vi "Scripting Mngr.vi"(0 "Path (dialog)":path, 1 "Mngr Action":T5, 3 "Main References":T4, 5 "Bottle X":T3, 7 "Drain X":T2, 9 "Well X":T1, 11 "error in (no error)":errorcluster, 12 "Script Choice":T6) -> (4 "selected path":path, 15 "error out":errorcluster)   [LabVIEW 2020]
uses:
  Script Mngr Script choice.ctl
  Script Mngr Action.ctl
  Main Refs.ctl
  Lib/Time/Bottles.ctl
  Drain Valve.ctl
  Lib/Time/Wells.ctl
  Hardware/Tricon Mngr.ctl
  Hardware/Tecan/Pump Control.ctl
  Pump Port.ctl
  Hardware/Tecan/Velocity Units.ctl
  Hardware/Valco Valve/Valco Valve Mngr Action.ctl
  Hardware/16CH Denkovi Mngr.ctl
  Hardware/Mot Stage Mngr.ctl
  Main Globals.vi
panel:
  in  "Pressure Valves X":bool[](array[boolean])
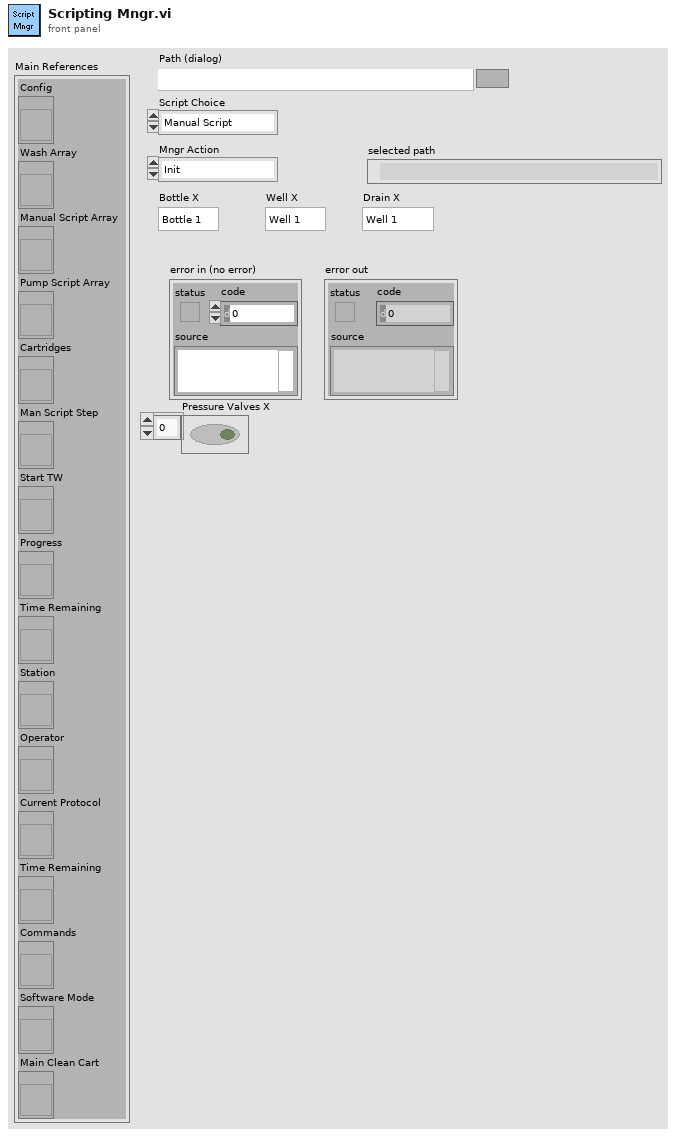
[diagram p1: front panel]
types:
  T1 = typedef "Wells.ctl" = enum16{"Well 1", "Well 2", "Well 3", "Well 4"}
  T2 = typedef "Drain Valve.ctl" = enum16{"Well 1", "Well 2", "Well 3", "Well 4", "Well X"}
  T3 = typedef "Bottles.ctl" = enum16{"Bottle 1", "Bottle 2", "Bottle 3", "H2O", "Waste"}
  T4 = typedef "Main Refs.ctl" = cluster{"Config":refnum<vi>, "Wash Array":refnum<vi>, "Manual Script Array":refnum<vi>, "Pump Script Array":refnum<vi>, "Cartridges":refnum<vi>, "Man Script Step":refnum<vi>, "Start TW":refnum<vi>, "Progress":refnum<vi>, "Time Remaining":refnum<vi>, "Station":refnum<vi>, "Operator":refnum<vi>, "Current Protocol":refnum<vi>, "Time Remaining":refnum<vi>, "Commands":refnum<vi>, "Software Mode":refnum<vi>, "Main Clean Cart":refnum<vi>}
  T5 = typedef "Script Mngr Action.ctl" = enum16{"Init", "Run Script", "Load Script", "Save Script", "Close"}
  T6 = typedef "Script Mngr Script choice.ctl" = enum16{"Manual Script", "Pump Script", "Wash Setup"}
  T7 = typedef "Pump Control.ctl" = cluster{"Syringe Pos":u32, "Rate":dbl, "Volume":dbl, "Valve":T8, "Action":enum32{"Withdraw", "Dispense", "Stop"}, "Move Type":enum32{"Abs", "Rel"}, "Init":bool, "Empty Syr.":bool, "Full Fill":bool, "Units":T9}
  T8 = typedef "Pump Port.ctl" = enum16{"Bottle 1", "Bottle 2", "Bottle 3", "Bottle 4", "Waste", "Well 1", "Well 2", "Well 3", "Well 4", "Bottle X", "Well X"}
  T9 = typedef "Velocity Units.ctl" = enum16{"ul/s", "ul/min"}
  T10 = typedef "Tricon Mngr.ctl" = enum16{"Init COM", "Set Config", "Init Pump", "Home", "Cmd", "Start Pump", "Set Valve", "Dispense", "Withdraw", "Status", "Close"}
  T11 = typedef "Mot Stage Mngr.ctl" = enum16{"Connect", "Init", "Status", "Send Cmd", "Current Pos", "Set Accel", "Set Max Vel", "Home", "Rel Move", "Abs Move", "Close"}
  T12 = typedef "16CH Denkovi Mngr.ctl" = enum16{"Search", "Init", "Set Peristaltic", "Set Pressure", "Set Vacuum", "Pres Vent&Close", "Vac Vent&Close", "Pres ON", "Vac ON", "Set All Relays", "Set One Relay", "Read Relays", "Close"}
  T13 = typedef "Valco Valve Mngr Action.ctl" = enum16{"Connect", "Init", "Cmd", "Set Valve", "Status", "Close"}
  T14 = typedef "Pump Script Step.ctl" = cluster{"Valve":enum16{"Valve 1", "Valve 2", "Valve 3", "Valve 4", "Valve 5", "Valve 6", "Valve 7", "Valve 8", "Valve 9"}, "Syr.Amount":dbl, "Syr.Rate":dbl, "move type":enum32{"rel", "abs"}, "direction":enum32{"withdraw", "dispense"}, "Delay(s)":dbl}
  T15 = enum16{"Valve 1", "Valve 2", "Valve 3", "Valve 4", "Valve 5", "Valve 6", "Valve 7", "Valve 8", "Valve 9"}
  T16 = typedef "Script Step.ctl" = cluster{"Step":dbl, "Step En":bool, "Valve":T8, "Syr.Amount":dbl, "Syr.Rate":dbl, "direction":enum32{"withdraw", "dispense"}, "Move Type":enum32{"Abs", "Rel"}, "Pump En":bool, "Drain Valve":T2, "Drain En":bool, "Peristaltic":bool, "Peristaltic En":bool, "Pres1":bool, "Pres2":bool, "Pres3":bool, "Pres4":bool, "Pressure En":bool, "Move Abs":dbl, "Motion En":bool, "Delay(s)":dbl, "Delay En":bool, "Use PresX":bool, "Vac1":bool, "Vac2":bool, "Vac3":bool, "Vac4":bool, "Use VacX":bool}
  T17 = typedef "Wash Step.ctl" = cluster{"Reagent":string, "Bottle":enum16{"Bottle 1", "Bottle 2", "Bottle 3", "Bottle 4"}, "Wash Time(s)":dbl, "Dwell Time(s)":dbl, "# of Rinses":i16}
  T18 = cluster{"negative limit switch":bool, "positive limit switch":bool, "home switch":bool, "position marker":bool, "device enable":bool, "quick stop":bool, "general purpose J":bool, "general purpose I":bool, "general purpose H":bool, "general purpose G":bool, "general purpose F":bool, "general purpose E":bool, "general purpose D":bool, "general purpose C":bool, "general purpose B":bool, "general purpose A":bool}
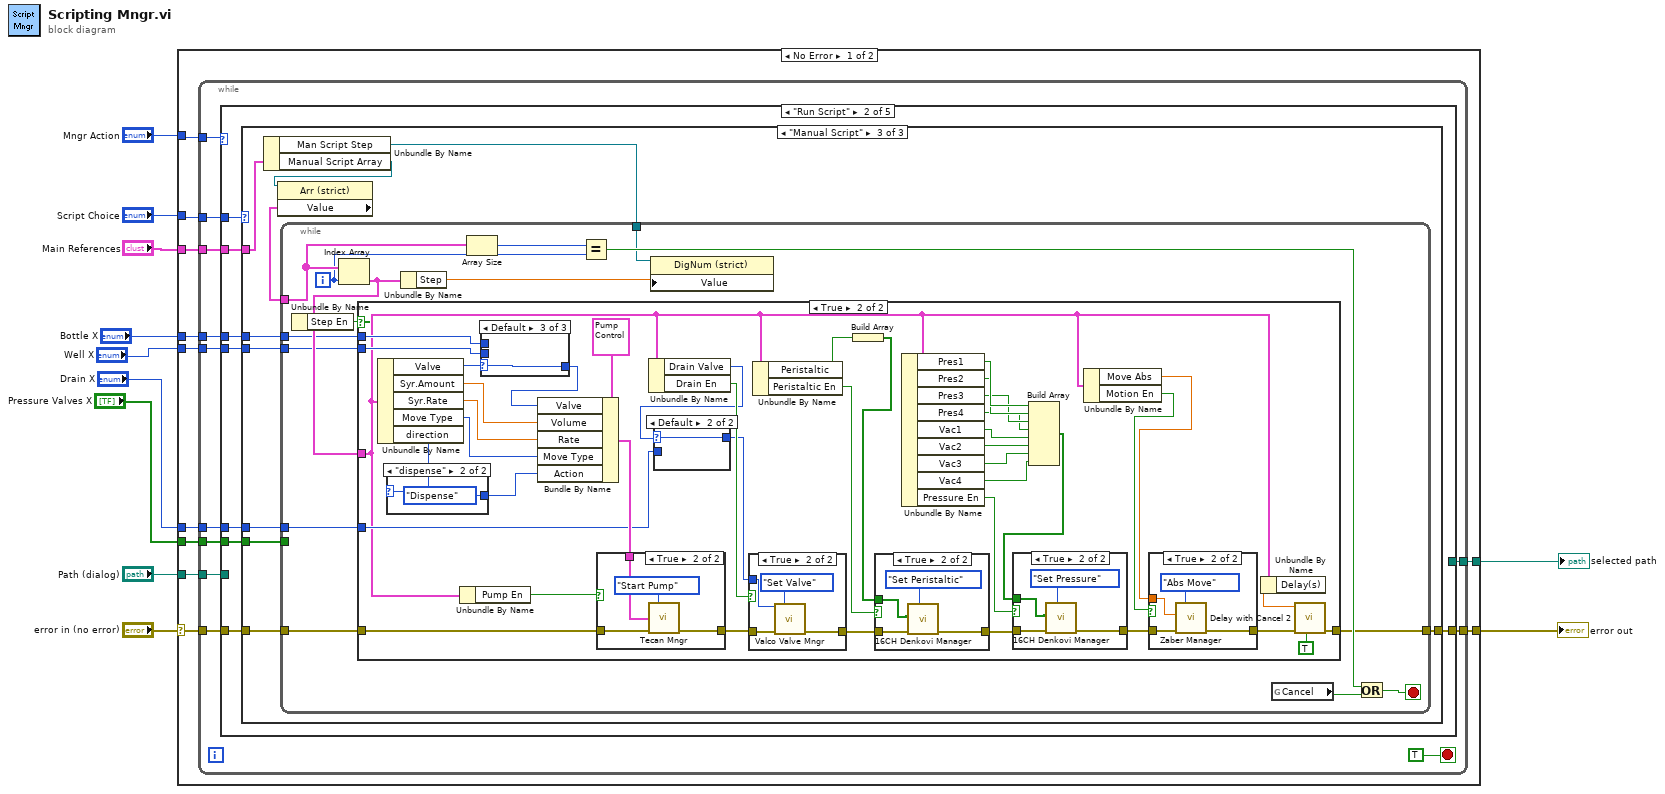
[diagram p0: block diagram]
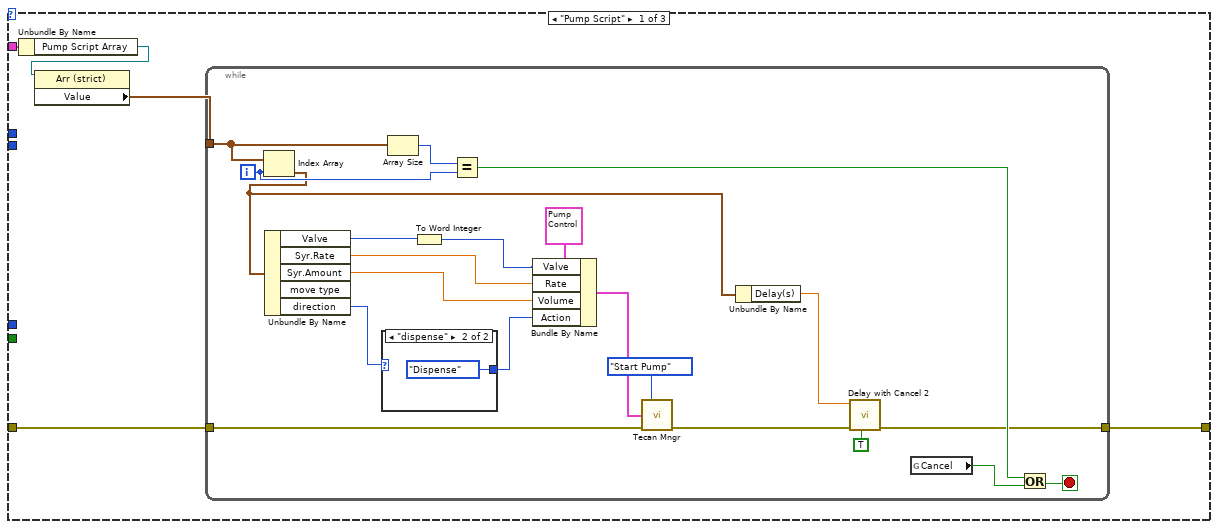
[diagram p3: hidden frame]
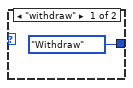
[diagram p4: hidden frame]
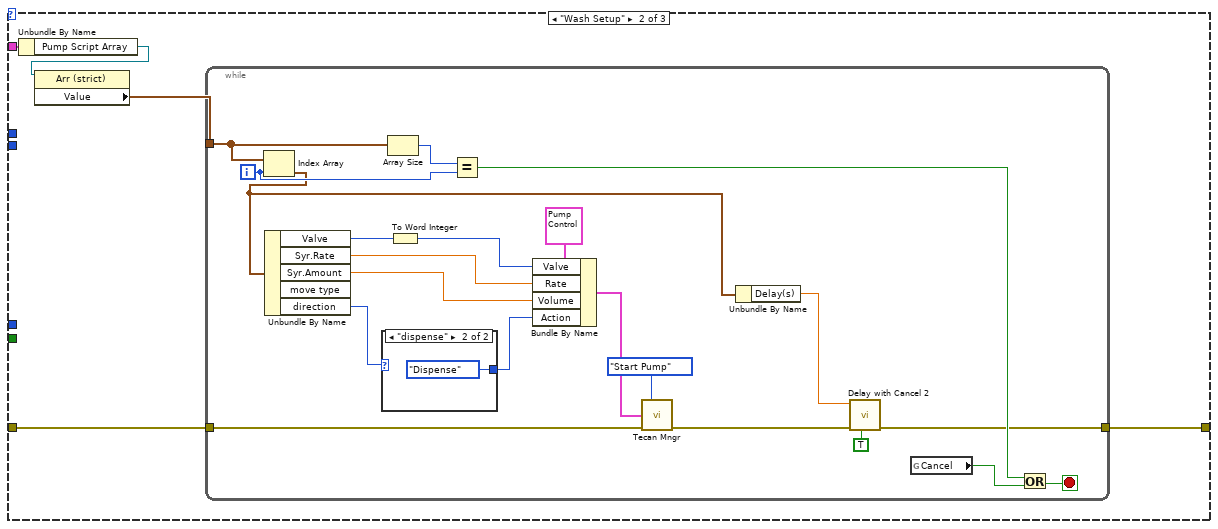
[diagram p5: hidden frame]
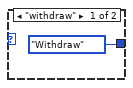
[diagram p6: hidden frame]
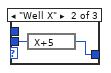
[diagram p10: hidden frame]
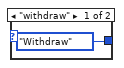
[diagram p16: hidden frame]
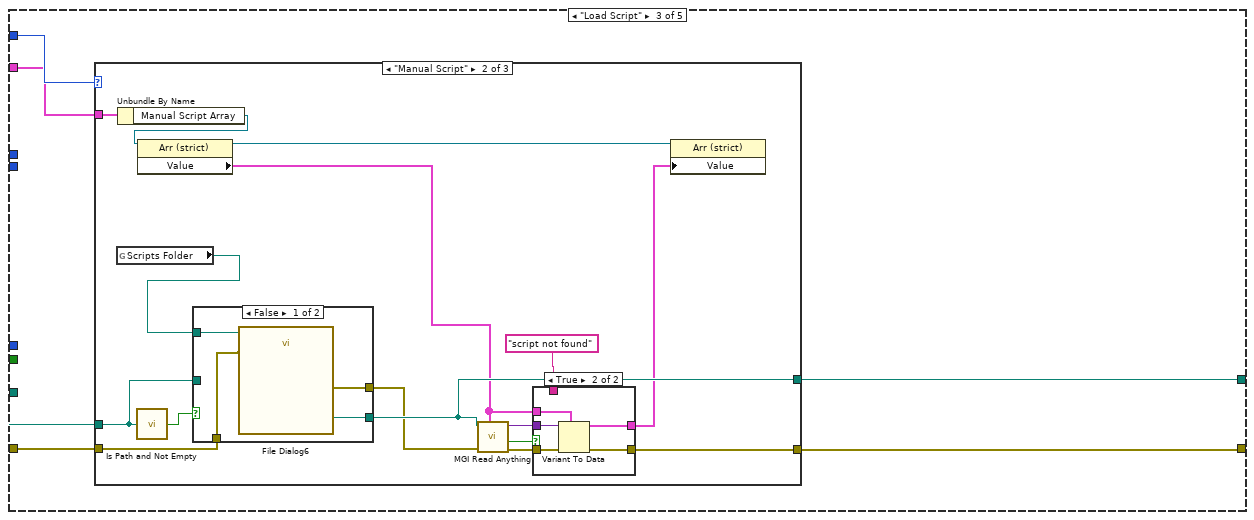
[diagram p17: hidden frame]
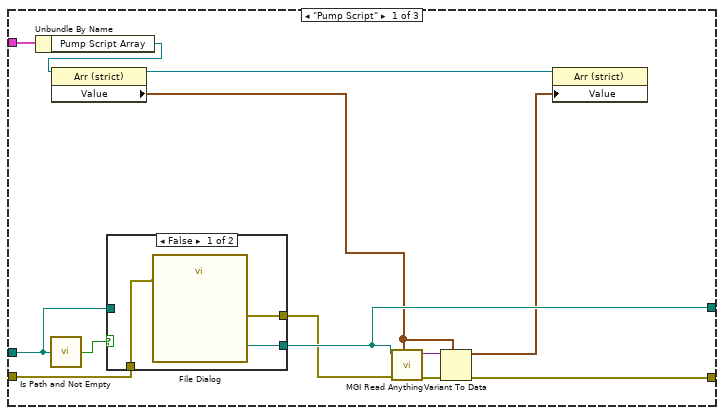
[diagram p18: hidden frame]
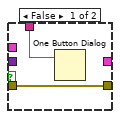
[diagram p20: hidden frame]
diagram:
  n1 = case shown="No Error" "error in (no error)" {
    selector: "error in (no error)" -> [w17 w310]
    tunnel: [w22 w310] -> w10
    tunnel: "Mngr Action" -> [w21 _]
    tunnel: "Script Choice" -> [w20 _]
    tunnel: "Path (dialog)" -> [w19 _]
    tunnel: [w18 _] -> w6
    tunnel: "Main References" -> [w16 _]
    tunnel: "Bottle X" -> [w15 _]
    tunnel: "Well X" -> [w14 _]
    tunnel: "Drain X" -> [w13 _]
    tunnel: "Pressure Valves X" -> [w12 _]
    frame No Error {
      n2 = while {
        tunnel: [w32] -> w22
        tunnel: w21 -> [w33]
        tunnel: w20 -> [w31]
        tunnel: w19 -> [w30]
        tunnel: [w29] -> w18
        tunnel: w17 -> [w28]
        tunnel: w16 -> [w27]
        tunnel: w15 -> [w26]
        tunnel: w14 -> [w25]
        tunnel: w13 -> [w24]
        tunnel: w12 -> [w23]
        stop <- TRUE stop-if-true
        n3 = case shown="\"Run Script\"" w33 {
          tunnel: w28 -> [w35 w42 w204 w275 w309]
          tunnel: [w35 w43 w203 w274 w309] -> w32
          tunnel: w31 -> [_ w41 w205 w276 _]
          tunnel: w30 -> [_ _ w202 w273 _]
          tunnel: [_ _ w201 w272 _] -> w29
          tunnel: w27 -> [_ w40 w200 w271 _]
          tunnel: w26 -> [_ w39 _ _ _]
          tunnel: w25 -> [_ w38 _ _ _]
          tunnel: w24 -> [_ w37 _ _ _]
          tunnel: w23 -> [_ w36 _ _ _]
          frame "Init" {
          }
          frame "Run Script" {
            n4 = case shown="\"Manual Script\"" w41 {
              tunnel: [w47 w75 w108] -> w43
              tunnel: w42 -> [w48 w76 w109]
              tunnel: w40 -> [w46 w74 w107]
              tunnel: w39 -> [_ _ w103]
              tunnel: w38 -> [_ _ w102]
              tunnel: w37 -> [_ _ w101]
              tunnel: w36 -> [_ _ w100]
              frame "Pump Script" {
                n5 = Unbundle By Name(w46) -> ("Pump Script Array"=w45:refnum<vi>)
                n6 = property class="Arr (strict)"(reference=w45) -> ("Value"=w44:T14[])  [unwired: 1 in, 2 out]
                n7 = while {
                  tunnel: w48 -> [w63]
                  tunnel: w44 -> [w68]
                  tunnel: [w53] -> w47
                  i -> [w66]
                  stop <- w69 stop-if-true
                  n8 = Index Array(array=w68, index=w66) -> (element=w56:T14)
                  n9 = Unbundle By Name(w56) -> ("Valve"=w50:T15, "Syr.Rate"=w60:dbl, "Syr.Amount"=w59:dbl, "direction"=w58:enum32{"withdraw", "dispense"})  [unwired: 1 out]
                  n10 = case shown="\"dispense\"" w58 {
                    tunnel: [enum32{"Withdraw", "Dispense", "Stop"}."Withdraw" ("Action") enum32{"Withdraw", "Dispense", "Stop"}."Dispense" ("Action")] -> w57
                    frame "withdraw" {
                    }
                    frame "dispense" {
                    }
                  }
                  n11 = Array Size(array=w68) -> (size(s)=w67:i32)
                  n12 = To Word Integer(number=w50) -> (16bit integer=w49:i16)
                  n13 = Equal?(x=w67, y=w66) -> (x = y?=w65:bool)
                  n14 = Bundle By Name(cluster=T7 {"Syringe Pos"=500, "Rate"=400.0, "Volume"=500.0, "Valve"=enum."Bottle 3", "Action"=enum."Dispense", "Move Type"=enum."Rel", "Init"=TRUE, "Empty Syr."=TRUE, "Full Fill"=TRUE, "Units"=enum."ul/s"} ("Pump Data"), "Valve"=w49, "Rate"=w60, "Volume"=w59, "Action"=w57) -> (w51:T7)
                  n15 = call "Tecan Mngr.vi"("Mngr Action"=Tricon_Mngr."Start Pump", "Pump Data"=w51, "error in (no error)"=w63) -> ("error out"=w55:errorcluster)  [unwired: 7 in, 5 out]
                  n16 = Unbundle By Name(w56) -> ("Delay(s)"=w54:dbl)
                  n17 = call "Delay with Cancel 2.vi"("Insert Error"=TRUE, "error in (no error)"=w55, "Delay(s)"=w54) -> ("error out"=w53:errorcluster)  [unwired: 7 in, 1 out]
                  n18 = global read "Main Globals.vi" "Cancel"() -> (w64:bool)
                  n19 = Or(x=w65, y=w64) -> (x .or. y?=w69:bool)
                }
              }
              frame "Wash Setup" {
                n20 = Unbundle By Name(w74) -> ("Pump Script Array"=w73:refnum<vi>)
                n21 = property class="Arr (strict)"(reference=w73) -> ("Value"=w72:T14[])  [unwired: 1 in, 2 out]
                n22 = while {
                  tunnel: w76 -> [w91]
                  tunnel: w72 -> [w96]
                  tunnel: [w81] -> w75
                  i -> [w94]
                  stop <- w97 stop-if-true
                  n23 = Index Array(array=w96, index=w94) -> (element=w84:T14)
                  n24 = Unbundle By Name(w84) -> ("Valve"=w79:T15, "Syr.Rate"=w88:dbl, "Syr.Amount"=w87:dbl, "direction"=w86:enum32{"withdraw", "dispense"})  [unwired: 1 out]
                  n25 = case shown="\"dispense\"" w86 {
                    tunnel: [enum32{"Withdraw", "Dispense", "Stop"}."Withdraw" ("Action") enum32{"Withdraw", "Dispense", "Stop"}."Dispense" ("Action")] -> w85
                    frame "withdraw" {
                    }
                    frame "dispense" {
                    }
                  }
                  n26 = Array Size(array=w96) -> (size(s)=w95:i32)
                  n27 = To Word Integer(number=w79) -> (16bit integer=w78:i16)
                  n28 = Equal?(x=w95, y=w94) -> (x = y?=w93:bool)
                  n29 = Bundle By Name(cluster=T7 {"Syringe Pos"=500, "Rate"=400.0, "Volume"=500.0, "Valve"=enum."Bottle 3", "Action"=enum."Dispense", "Move Type"=enum."Rel", "Init"=TRUE, "Empty Syr."=TRUE, "Full Fill"=TRUE, "Units"=enum."ul/s"} ("Pump Data"), "Valve"=w78, "Rate"=w88, "Volume"=w87, "Action"=w85) -> (w77:T7)
                  n30 = call "Tecan Mngr.vi"("Mngr Action"=Tricon_Mngr."Start Pump", "Pump Data"=w77, "error in (no error)"=w91) -> ("error out"=w83:errorcluster)  [unwired: 7 in, 5 out]
                  n31 = Unbundle By Name(w84) -> ("Delay(s)"=w82:dbl)
                  n32 = call "Delay with Cancel 2.vi"("Insert Error"=TRUE, "error in (no error)"=w83, "Delay(s)"=w82) -> ("error out"=w81:errorcluster)  [unwired: 7 in, 1 out]
                  n33 = global read "Main Globals.vi" "Cancel"() -> (w92:bool)
                  n34 = Or(x=w93, y=w92) -> (x .or. y?=w97:bool)
                }
              }
              frame "Manual Script" {
                n35 = Unbundle By Name(w107) -> ("Man Script Step"=w104:refnum<vi>, "Manual Script Array"=w106:refnum<vi>)
                n36 = property class="Arr (strict)"(reference=w106) -> ("Value"=w105:T16[])  [unwired: 1 in, 2 out]
                n37 = while {
                  tunnel: w109 -> [w120]
                  tunnel: w105 -> [w124]
                  tunnel: [w119] -> w108
                  tunnel: w104 -> [w116]
                  tunnel: w103 -> [w114]
                  tunnel: w102 -> [w113]
                  tunnel: w101 -> [w112]
                  tunnel: w100 -> [_]
                  i -> [w122]
                  stop <- w110 stop-if-true
                  n38 = Index Array(array=w124, index=w122) -> (element=w117:T16)
                  n39 = Unbundle By Name(w117) -> ("Step En"=w118:bool)
                  n40 = case shown="True" w118 {
                    tunnel: w120 -> [w125 w166]
                    tunnel: [w125 w162] -> w119
                    tunnel: w117 -> [_ w131]
                    tunnel: w114 -> [_ w137]
                    tunnel: w113 -> [_ w135]
                    tunnel: w112 -> [_ w133]
                    frame False {
                    }
                    frame True {
                      n41 = Unbundle By Name(w131) -> ("Valve"=w138:T8, "Syr.Amount"=w160:dbl, "Syr.Rate"=w159:dbl, "Move Type"=w139:enum32{"Abs", "Rel"}, "direction"=w140:enum32{"withdraw", "dispense"})
                      n42 = case shown="\"dispense\"" w140 {
                        tunnel: [enum32{"Withdraw", "Dispense", "Stop"}."Withdraw" ("Action") enum32{"Withdraw", "Dispense", "Stop"}."Dispense" ("Action")] -> w141
                        frame "withdraw" {
                        }
                        frame "dispense" {
                        }
                      }
                      n43 = Unbundle By Name(w131) -> ("Pump En"=w158:bool)
                      n44 = case shown="Default" w138 {
                        selector: w138 -> [_ _ w172]
                        tunnel: w137 -> [w169 _ _]
                        tunnel: [w169 w170 w172] -> w136
                        tunnel: w135 -> [_ w171 _]
                        frame "Bottle X" {
                        }
                        frame "Well X" {
                          n45 = expression code="X+5"(w171) -> (w170:T1)
                        }
                        frame Default {
                        }
                      }
                      n46 = Bundle By Name(cluster=T7 {"Syringe Pos"=500, "Rate"=400.0, "Volume"=500.0, "Valve"=enum."Bottle 3", "Action"=enum."Dispense", "Move Type"=enum."Rel", "Init"=TRUE, "Empty Syr."=TRUE, "Full Fill"=TRUE, "Units"=enum."ul/s"} ("Pump Data"), "Valve"=w136, "Volume"=w160, "Rate"=w159, "Move Type"=w139, "Action"=w141) -> (w164:T7)
                      n47 = case shown="True" w158 {
                        tunnel: w166 -> [w193 w197]
                        tunnel: w164 -> [_ w194]
                        tunnel: [w193 w195] -> w157
                        frame False {
                        }
                        frame True {
                          n48 = call "Tecan Mngr.vi"("Mngr Action"=Tricon_Mngr."Start Pump", "Pump Data"=w194, "error in (no error)"=w197) -> ("error out"=w195:errorcluster)  [unwired: 7 in, 5 out]
                        }
                      }
                      n49 = Unbundle By Name(w131) -> ("Drain Valve"=w134:T2, "Drain En"=w156:bool)
                      n50 = case shown="Default" w134 {
                        selector: w134 -> [_ w168]
                        tunnel: w133 -> [w167 _]
                        tunnel: [w167 w168] -> w132
                        frame "Well X" {
                        }
                        frame Default {
                        }
                      }
                      n51 = case shown="True" w156 {
                        tunnel: w157 -> [w188 w192]
                        tunnel: [w188 w191] -> w155
                        tunnel: w132 -> [_ w190]
                        frame False {
                        }
                        frame True {
                          n52 = call "Valco Valve Mngr.vi"("Valve"=w190, "Mngr Action"=Valco_Valve_Mngr_Action."Set Valve", "error in (no error)"=w192) -> ("error out"=w191:errorcluster)  [unwired: 8 in, 4 out]
                        }
                      }
                      n53 = Unbundle By Name(w131) -> ("Peristaltic"=w153:bool, "Peristaltic En"=w154:bool)
                      n54 = Build Array(w153) -> (w152:bool[])
                      n55 = case shown="True" w154 {
                        tunnel: w155 -> [w183 w187]
                        tunnel: [w183 w186] -> w146
                        tunnel: w152 -> [_ w184]
                        frame False {
                        }
                        frame True {
                          n56 = call "16CH Denkovi Manager.vi"("Action"=16CH_Denkovi_Mngr."Set Peristaltic", "error in (no error)"=w187, "Relays In"=w184) -> ("error out"=w186:errorcluster)  [unwired: 6 in, 2 out]
                        }
                      }
                      n57 = Unbundle By Name(w131) -> ("Pres1"=w151:bool, "Pres2"=w150:bool, "Pres3"=w149:bool, "Pres4"=w148:bool, "Vac1"=w130:bool, "Vac2"=w129:bool, "Vac3"=w127:bool, "Vac4"=w128:bool, "Pressure En"=w126:bool)
                      n58 = Build Array(w151, w150, w149, w148, w130, w129, w127, w128) -> (w147:bool[])
                      n59 = case shown="True" w126 {
                        tunnel: w146 -> [w178 w182]
                        tunnel: [w178 w181] -> w145
                        tunnel: w147 -> [_ w179]
                        frame False {
                        }
                        frame True {
                          n60 = call "16CH Denkovi Manager.vi"("Action"=16CH_Denkovi_Mngr."Set Pressure", "error in (no error)"=w182, "Relays In"=w179) -> ("error out"=w181:errorcluster)  [unwired: 6 in, 2 out]
                        }
                      }
                      n61 = Unbundle By Name(w131) -> ("Move Abs"=w143:dbl, "Motion En"=w144:bool)
                      n62 = case shown="True" w144 {
                        tunnel: w145 -> [w173 w177]
                        tunnel: [w173 w176] -> w142
                        tunnel: w143 -> [_ w174]
                        frame False {
                        }
                        frame True {
                          n63 = call "Zaber Manager.vi"("Action"=Mot_Stage_Mngr."Abs Move", "Value"=w174, "error in (no error)"=w177) -> ("error out"=w176:errorcluster)  [unwired: 6 in, 6 out]
                        }
                      }
                      n64 = Unbundle By Name(w131) -> ("Delay(s)"=w163:dbl)
                      n65 = call "Delay with Cancel 2.vi"("Insert Error"=TRUE, "error in (no error)"=w142, "Delay(s)"=w163) -> ("error out"=w162:errorcluster)  [unwired: 7 in, 1 out]
                    }
                  }
                  n66 = Unbundle By Name(w117) -> ("Step"=w115:dbl)
                  n67 = Array Size(array=w124) -> (size(s)=w123:i32)
                  n68 = Equal?(x=w123, y=w122) -> (x = y?=w121:bool)
                  n69 = property class="DigNum (strict)"(reference=w116, "Value"=w115) -> ()  [unwired: 1 in, 2 out]
                  n70 = global read "Main Globals.vi" "Cancel"() -> (w111:bool)
                  n71 = Or(x=w121, y=w111) -> (x .or. y?=w110:bool)
                }
              }
            }
          }
          frame "Load Script" {
            n72 = case shown="\"Manual Script\"" w205 {
              tunnel: w204 -> [w211 w232 w258]
              tunnel: [w216 w237 w263] -> w203
              tunnel: w202 -> [w213 w234 w260]
              tunnel: [w214 w235 w261] -> w201
              tunnel: w200 -> [w209 w230 w256]
              frame "Pump Script" {
                n73 = Unbundle By Name(w209) -> ("Pump Script Array"=w210:refnum<vi>)
                n74 = call <vilib>:"Is Path and Not Empty.vi"("path"=w213) -> ("Is Path and Not Empty?"=w215:bool)  [unwired: 4 in]
                n75 = property class="Arr (strict)"(reference=w210) -> (reference out=w207:refnum<vi>, "Value"=w208:T14[])  [unwired: 1 in, 1 out]
                n76 = case shown="False" w215 {
                  tunnel: [w221 w223] -> w214
                  tunnel: w213 -> [_ w223]
                  tunnel: [w220 w222] -> w212
                  tunnel: w211 -> [w219 w222]
                  frame False {
                    n77 = call "File Dialog"("error in"=w219) -> ("selected path"=w221:path, "error out"=w220:errorcluster)  [unwired: 11 in, 2 out]
                  }
                  frame True {
                  }
                }
                n78 = call <userlib>:"MGI Read Anything.vi"("Type of Anything"=w208, "Error In"=w212, "Path (dialog)"=w214) -> ("Error Out"=w218:errorcluster, "Anything"=w217:variant)  [unwired: 5 in, 2 out]
                n79 = Variant To Data(error in=w218, type=w208, Variant=w217) -> (data=w206:T14[], error out=w216:errorcluster)
                n80 = property class="Arr (strict)"(reference=w207, "Value"=w206) -> ()  [unwired: 1 in, 2 out]
              }
              frame "Manual Script" {
                n81 = global read "Main Globals.vi" "Scripts Folder"() -> (w226:path)
                n82 = Unbundle By Name(w230) -> ("Manual Script Array"=w231:refnum<vi>)
                n83 = call <vilib>:"Is Path and Not Empty.vi"("path"=w234) -> ("Is Path and Not Empty?"=w236:bool)  [unwired: 4 in]
                n84 = property class="Arr (strict)"(reference=w231) -> (reference out=w228:refnum<vi>, "Value"=w229:T16[])  [unwired: 1 in, 1 out]
                n85 = case shown="False" w236 {
                  tunnel: [w250 w252] -> w235
                  tunnel: w234 -> [_ w252]
                  tunnel: [w249 w251] -> w233
                  tunnel: w232 -> [w248 w251]
                  tunnel: w226 -> [w247 _]
                  frame False {
                    n86 = call "File Dialog6"("start path"=w247, "error in"=w248) -> ("selected path"=w250:path, "error out"=w249:errorcluster)  [unwired: 10 in, 2 out]
                  }
                  frame True {
                  }
                }
                n87 = call <userlib>:"MGI Read Anything.vi"("Type of Anything"=w229, "Error In"=w233, "Path (dialog)"=w235) -> ("Error Out"=w239:errorcluster, "Found?"=w225:bool, "Anything"=w238:variant)  [unwired: 5 in, 1 out]
                n88 = case shown="True" w225 {
                  tunnel: w239 -> [w240 w246]
                  tunnel: w238 -> [_ w245]
                  tunnel: [w240 w244] -> w237
                  tunnel: w229 -> [_ w243]
                  tunnel: [_ w242] -> w227
                  tunnel: "script not found" ("message") -> [w241 _]
                  frame False {
                    n89 = One Button Dialog(message=w241) -> ()  [unwired: 1 in, 1 out]
                  }
                  frame True {
                    n90 = Variant To Data(error in=w246, type=w243, Variant=w245) -> (data=w242:T16[], error out=w244:errorcluster)
                  }
                }
                n91 = property class="Arr (strict)"(reference=w228, "Value"=w227) -> ()  [unwired: 1 in, 2 out]
              }
              frame "Wash Setup" {
                n92 = call <vilib>:"Is Path and Not Empty.vi"("path"=w260) -> ("Is Path and Not Empty?"=w262:bool)  [unwired: 4 in]
                n93 = Unbundle By Name(w256) -> ("Wash Array"=w257:refnum<vi>)
                n94 = property class="Arr (strict)"(reference=w257) -> (reference out=w254:refnum<vi>, "Value"=w255:T17[])  [unwired: 1 in, 1 out]
                n95 = case shown="False" w262 {
                  tunnel: [w268 w270] -> w261
                  tunnel: w260 -> [_ w270]
                  tunnel: [w267 w269] -> w259
                  tunnel: w258 -> [w266 w269]
                  frame False {
                    n96 = call "File Dialog5"("error in"=w266) -> ("selected path"=w268:path, "error out"=w267:errorcluster)  [unwired: 11 in, 2 out]
                  }
                  frame True {
                  }
                }
                n97 = call <userlib>:"MGI Read Anything.vi"("Type of Anything"=w255, "Error In"=w259, "Path (dialog)"=w261) -> ("Error Out"=w265:errorcluster, "Anything"=w264:variant)  [unwired: 5 in, 2 out]
                n98 = Variant To Data(error in=w265, type=w255, Variant=w264) -> (data=w253:T17[], error out=w263:errorcluster)
                n99 = property class="Arr (strict)"(reference=w254, "Value"=w253) -> ()  [unwired: 1 in, 2 out]
              }
            }
          }
          frame "Save Script" {
            n100 = case shown="\"Manual Script\"" w276 {
              tunnel: w275 -> [w281 w291 w302]
              tunnel: [w284 w294 w305] -> w274
              tunnel: w273 -> [w282 w292 w303]
              tunnel: [w280 w290 w301] -> w272
              tunnel: w271 -> [w278 w288 w299]
              frame "Pump Script" {
                n101 = call <vilib>:"Is Path and Not Empty.vi"("path"=w282) -> ("Is Path and Not Empty?"=w283:bool)  [unwired: 4 in]
                n102 = Unbundle By Name(w278) -> ("Pump Script Array"=w279:refnum<vi>)
                n103 = property class="Arr (strict)"(reference=w279) -> ("Value"=w277:T14[])  [unwired: 1 in, 2 out]
                n104 = case shown="False" w283 {
                  tunnel: [w285 w286] -> w280
                  tunnel: w282 -> [_ w286]
                  frame False {
                    n105 = call "File Dialog2"() -> ("selected path"=w285:path)  [unwired: 12 in, 3 out]
                  }
                  frame True {
                  }
                }
                n106 = call <userlib>:"MGI Write Anything.vi"("Error In"=w281, "Anything"=w277, "Path (dialog)"=w280) -> ("Error Out"=w284:errorcluster)  [unwired: 6 in, 2 out]
              }
              frame "Wash Setup" {
                n107 = call <vilib>:"Is Path and Not Empty.vi"("path"=w292) -> ("Is Path and Not Empty?"=w293:bool)  [unwired: 4 in]
                n108 = Unbundle By Name(w288) -> ("Wash Array"=w289:refnum<vi>)
                n109 = property class="Arr (strict)"(reference=w289) -> ("Value"=w287:T17[])  [unwired: 1 in, 2 out]
                n110 = case shown="False" w293 {
                  tunnel: [w295 w296] -> w290
                  tunnel: w292 -> [_ w296]
                  frame False {
                    n111 = call "File Dialog3"() -> ("selected path"=w295:path)  [unwired: 12 in, 3 out]
                  }
                  frame True {
                  }
                }
                n112 = call <userlib>:"MGI Write Anything.vi"("Error In"=w291, "Anything"=w287, "Path (dialog)"=w290) -> ("Error Out"=w294:errorcluster)  [unwired: 6 in, 2 out]
              }
              frame "Manual Script" {
                n113 = Unbundle By Name(w299) -> ("Manual Script Array"=w300:refnum<vi>)
                n114 = call <vilib>:"Is Path and Not Empty.vi"("path"=w303) -> ("Is Path and Not Empty?"=w304:bool)  [unwired: 4 in]
                n115 = global read "Main Globals.vi" "Scripts Folder"() -> (w297:path)
                n116 = property class="Arr (strict)"(reference=w300) -> ("Value"=w298:T16[])  [unwired: 1 in, 2 out]
                n117 = case shown="False" w304 {
                  tunnel: [w307 w308] -> w301
                  tunnel: w303 -> [_ w308]
                  tunnel: w297 -> [w306 _]
                  frame False {
                    n118 = call "File Dialog4"("start path"=w306) -> ("selected path"=w307:path)  [unwired: 11 in, 3 out]
                  }
                  frame True {
                  }
                }
                n119 = call <userlib>:"MGI Write Anything.vi"("Error In"=w302, "Anything"=w298, "Path (dialog)"=w301) -> ("Error Out"=w305:errorcluster)  [unwired: 6 in, 2 out]
              }
            }
          }
          frame "Close" {
          }
        }
      }
    }
    frame Error {
      (unwired) T18 {"negative limit switch"=FALSE, "positive limit switch"=FALSE, "home switch"=FALSE, "position marker"=FALSE, "device enable"=FALSE, "quick stop"=FALSE, "general purpose J"=FALSE, "general purpose I"=FALSE, "general purpose H"=FALSE, "general purpose G"=FALSE, "general purpose F"=FALSE, "general purpose E"=FALSE, "general purpose D"=FALSE, "general purpose C"=FALSE, "general purpose B"=FALSE, "general purpose A"=FALSE} ("digital inputs")
    }
  }
  "error out" <- w10
  "selected path" <- w6
